vi "get.Bytes.vi"(8 "error in (no error)":errorcluster, 11 "PitchMessage in":refnum<class "PitchMessage.lvclass">) -> (0 "error out":errorcluster, 2 "Bytes.Out":u8[](array[numeric]) format="%.0x", 3 "PitchMessage out":refnum<class "PitchMessage.lvclass">)   [LabVIEW 2022 SP3, in "PitchMessage.lvclass"]
uses:
  PitchMessage.lvclass
  PitchMessage.lvclass/PitchMessage.ctl
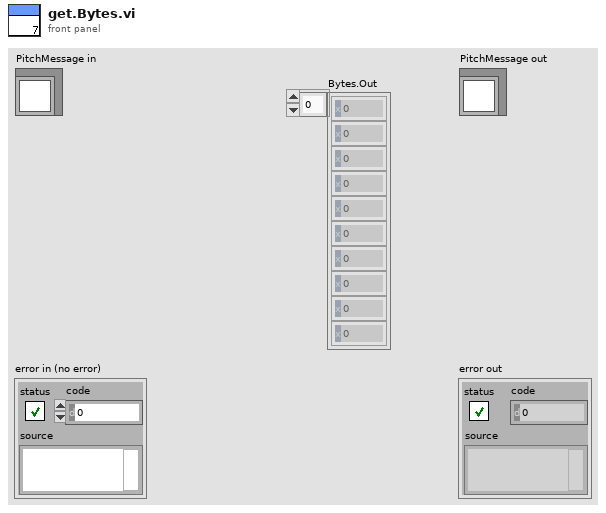
[diagram p1: front panel]
types:
  T1 = typedef "FieldValue.ctl" = variant
  T2 = typedef "FieldSpec.ctl" = cluster{"Name":string, "Offset":i32, "Length":i32, "FieldType":enum16{"Alphanumeric", "Binary", "BinaryLongPrice", "BinaryShortPrice", "BitField", "PrintableAscii", "Value"}, "FieldValue":variant}
  T3 = enum16{"Alphanumeric", "Binary", "BinaryLongPrice", "BinaryShortPrice", "BitField", "PrintableAscii", "Value"}
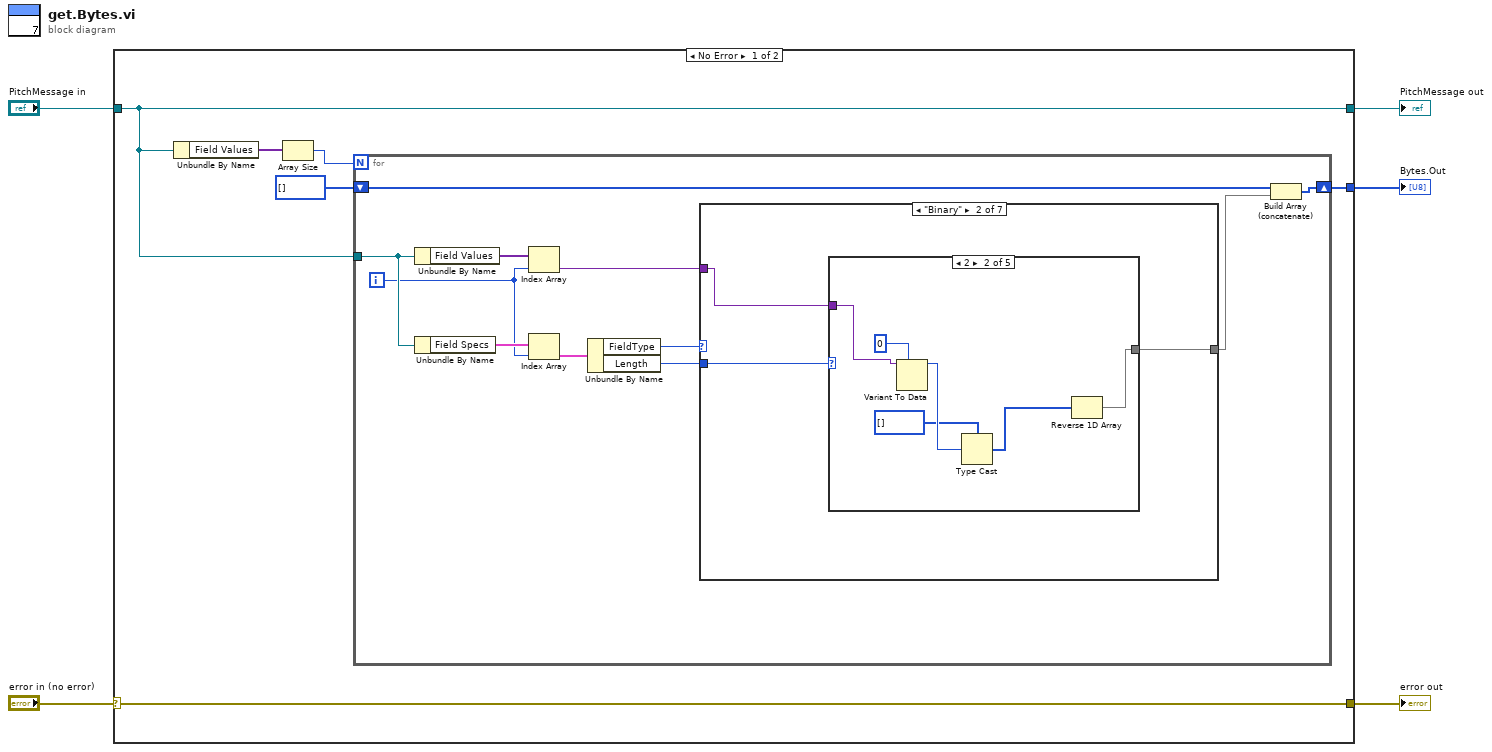
[diagram p0: block diagram]
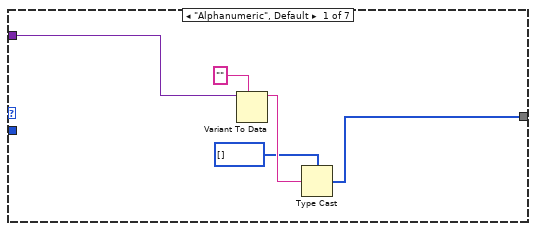
[diagram p2: hidden frame]
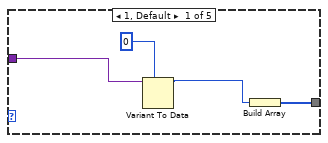
[diagram p3: hidden frame]
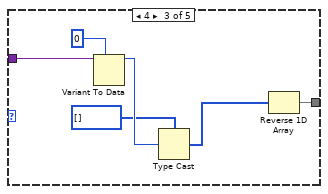
[diagram p4: hidden frame]
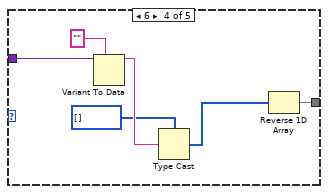
[diagram p5: hidden frame]
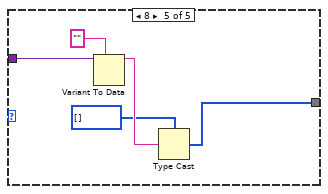
[diagram p6: hidden frame]
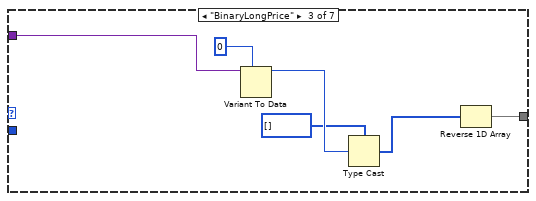
[diagram p7: hidden frame]
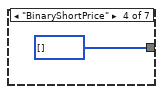
[diagram p8: hidden frame]
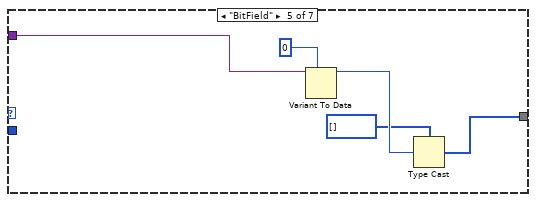
[diagram p9: hidden frame]
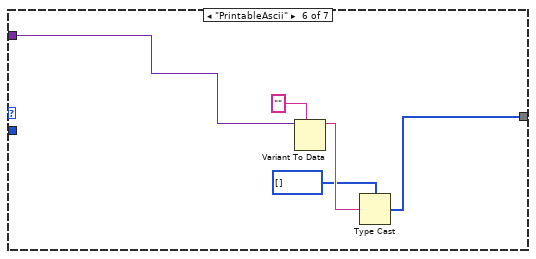
[diagram p10: hidden frame]
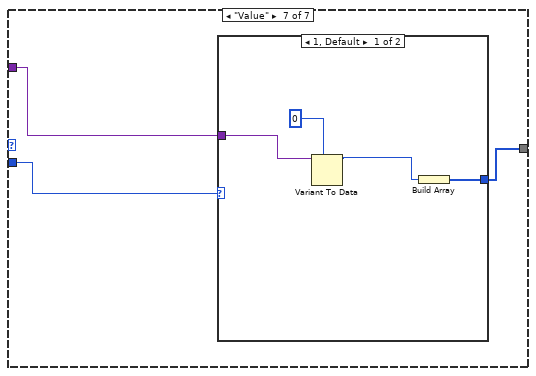
[diagram p11: hidden frame]
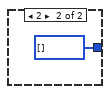
[diagram p12: hidden frame]
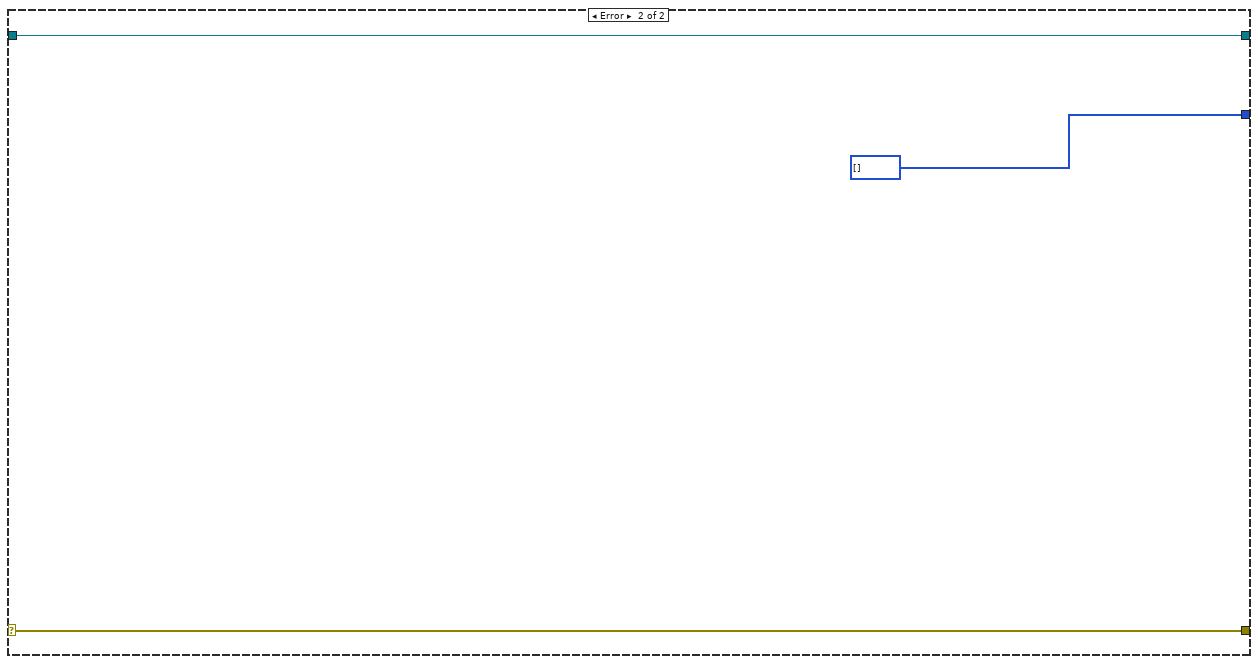
[diagram p13: hidden frame]
diagram:
  n1 = case shown="No Error" "error in (no error)" {
    selector: "error in (no error)" -> [w11 w85]
    tunnel: [w11 w85] -> w4
    tunnel: [w7 w84] -> w2
    tunnel: "PitchMessage in" -> [w7 w84]
    tunnel: [w9 u8[] []] -> w1
    frame No Error {
      n2 = Unbundle By Name(w7) -> ("Field Values"=w6:T1[])
      n3 = Array Size(array=w6) -> (size(s)=w8:i32)
      n4 = for {
        N: w8 -> [_]
        tunnel: w7 -> [w21]
        shift-right: [w14] -> w9
        shift-left: u8[] [] -> [w15]
        i -> [w12]
        n5 = Unbundle By Name(w21) -> ("Field Values"=w22:T1[])
        n6 = Unbundle By Name(w21) -> ("Field Specs"=w20:T2[])
        n7 = Index Array(array=w22, index=w12) -> (element=w16:T1)
        n8 = Index Array(array=w20, index=w12) -> (element=w19:T2)
        n9 = Unbundle By Name(w19) -> ("FieldType"=w18:T3, "Length"=w17:i32)
        n10 = case shown="\"Binary\"" w18 {
          tunnel: w17 -> [_ w30 _ _ _ _ w76]
          tunnel: w16 -> [w24 w29 w60 _ w65 w70 w77]
          tunnel: [w23 w28 w58 u8[] [] w66 w71 w75] -> w13
          frame "Alphanumeric", Default {
            n11 = Variant To Data(type="", Variant=w24) -> (data=w26:string)  [unwired: 1 in, 1 out]
            n12 = Type Cast(type=u8[] [], x=w26) -> (*(type *) &x=w23:u8[])
          }
          frame "Binary" {
            n13 = case shown="2" w30 {
              tunnel: w29 -> [w34 w35 w45 w51 w56]
              tunnel: [w31 w36 w41 w47 w53] -> w28
              frame 1, Default {
                n14 = Variant To Data(type=u8 0, Variant=w34) -> (data=w32:u8)  [unwired: 1 in, 1 out]
                n15 = Build Array(w32) -> (w31:u8[])
              }
              frame 2 {
                n16 = Variant To Data(type=u16 0, Variant=w35) -> (data=w39:u16)  [unwired: 1 in, 1 out]
                n17 = Type Cast(type=u8[] [], x=w39) -> (*(type *) &x=w37:u8[])
                n18 = Reverse 1D Array(array=w37) -> (reversed array=w36:u8[])
              }
              frame 4 {
                n19 = Variant To Data(type=u32 0, Variant=w45) -> (data=w44:u32)  [unwired: 1 in, 1 out]
                n20 = Type Cast(type=u8[] [], x=w44) -> (*(type *) &x=w42:u8[])
                n21 = Reverse 1D Array(array=w42) -> (reversed array=w41:u8[])
              }
              frame 6 {
                n22 = Variant To Data(type="", Variant=w51) -> (data=w50:string)  [unwired: 1 in, 1 out]
                n23 = Type Cast(type=u8[] [], x=w50) -> (*(type *) &x=w48:u8[])
                n24 = Reverse 1D Array(array=w48) -> (reversed array=w47:u8[])
              }
              frame 8 {
                n25 = Variant To Data(type="", Variant=w56) -> (data=w55:string)  [unwired: 1 in, 1 out]
                n26 = Type Cast(type=u8[] [], x=w55) -> (*(type *) &x=w53:u8[])
              }
            }
          }
          frame "BinaryLongPrice" {
            n27 = Variant To Data(type=u64 0, Variant=w60) -> (data=w63:u64)  [unwired: 1 in, 1 out]
            n28 = Type Cast(type=u8[] [], x=w63) -> (*(type *) &x=w59:u8[])
            n29 = Reverse 1D Array(array=w59) -> (reversed array=w58:u8[])
          }
          frame "BinaryShortPrice" {
          }
          frame "BitField" {
            n30 = Variant To Data(type=u8 0, Variant=w65) -> (data=w69:u8)  [unwired: 1 in, 1 out]
            n31 = Type Cast(type=u8[] [], x=w69) -> (*(type *) &x=w66:u8[])
          }
          frame "PrintableAscii" {
            n32 = Variant To Data(type="", Variant=w70) -> (data=w73:string)  [unwired: 1 in, 1 out]
            n33 = Type Cast(type=u8[] [], x=w73) -> (*(type *) &x=w71:u8[])
          }
          frame "Value" {
            n34 = case shown="1, Default" w76 {
              tunnel: w77 -> [w81 _]
              tunnel: [w78 u8[] []] -> w75
              frame 1, Default {
                n35 = Variant To Data(type=u8 0, Variant=w81) -> (data=w79:u8)  [unwired: 1 in, 1 out]
                n36 = Build Array(w79) -> (w78:u8[])
              }
              frame 2 {
              }
            }
          }
        }
        n37 = Build Array (concatenate)(w15, w13) -> (w14:u8[])
      }
    }
    frame Error {
    }
  }
  "error out" <- w4
  "PitchMessage out" <- w2
  "Bytes.Out" <- w1
